vi "generateSquare_match.vi"(8 "Match rate (0-1)":sgl min=0 max=1, 9 "match":i32) -> (2 "new match":i32, 3 "Match":bool)   [LabVIEW 2020]
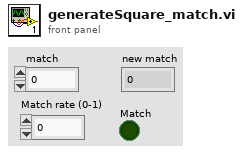
[diagram p1: front panel]
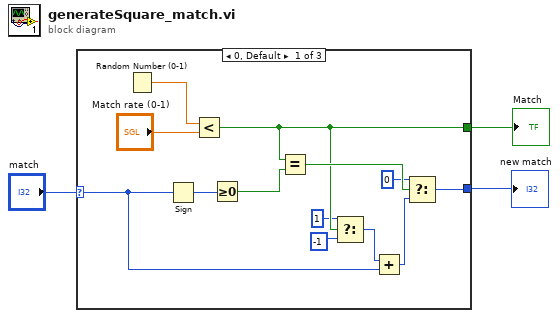
[diagram p0: block diagram]
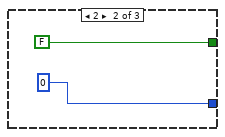
[diagram p2: hidden frame]
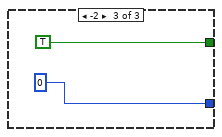
[diagram p3: hidden frame]
diagram:
  n1 = case shown="0, Default" "match" {
    selector: "match" -> [w6 _ _]
    tunnel: [w10 FALSE TRUE] -> w1
    tunnel: [w4 0 0] -> w2
    frame 0, Default {
      n2 = Random Number (0-1)() -> (number: 0 to 1=w15:dbl)
      n3 = Sign(1:w6) -> (0:w14:i32)
      n4 = Less?(x=w15, y="Match rate (0-1)") -> (x < y?=w10:bool)
      n5 = Greater Or Equal To 0?(x=w14) -> (x >= 0?=w13:bool)
      n6 = Equal?(x=w10, y=w13) -> (x = y?=w12:bool)
      n7 = Select(t=1, s=w10, f=-1) -> (s? t:f=w7:i32)
      n8 = Add(x=w7, y=w6) -> (x+y=w5:i32)
      n9 = Select(t=0, s=w12, f=w5) -> (s? t:f=w4:i32)
    }
    frame 2 {
    }
    frame -2 {
    }
  }
  "new match" <- w2
  "Match" <- w1
